vi "stop_device.vi"(8 "错误输入（无错误）":errorcluster) -> (0 "错误输出":errorcluster)   [LabVIEW 2013]
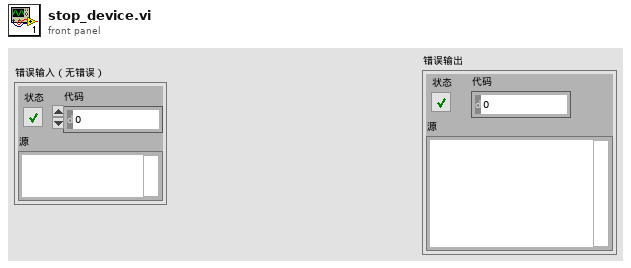
[diagram p1: front panel]
types:
  T1 = cluster{"cmd":string, "channel":i32, "value":dbl, "on/off":bool, "return value":refnum<vi>}
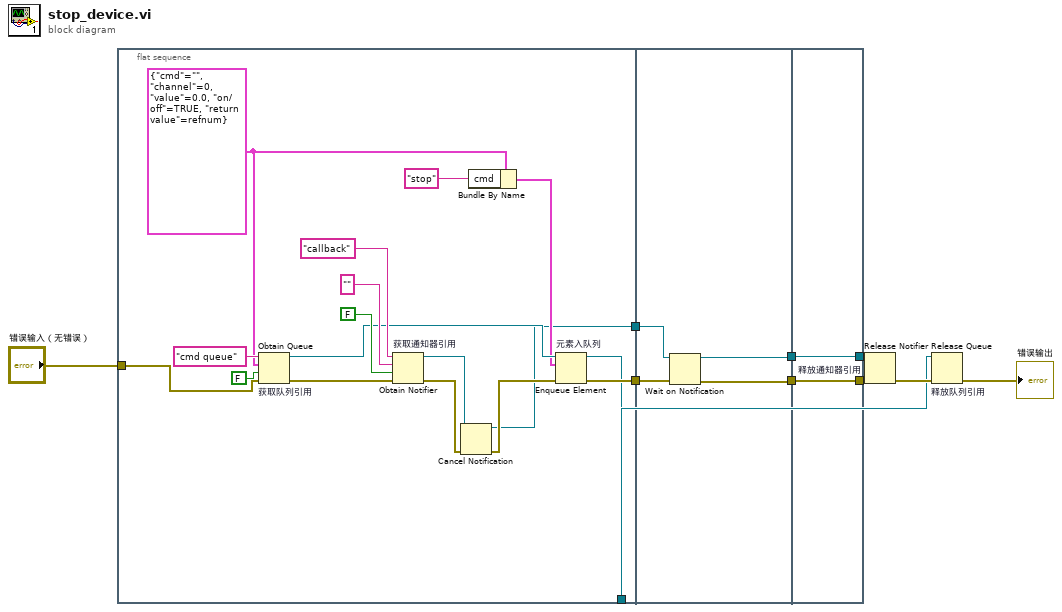
[diagram p0: block diagram]
diagram:
  n1 = flat-sequence {
    tunnel: [w11] -> w10
    tunnel: [w17] -> w5
    tunnel: [w16] -> w2
    tunnel: "错误输入（无错误）" -> [w15]
    tunnel: w10 -> [w31]
    tunnel: [w28] -> w9
    tunnel: [w29] -> w7
    tunnel: w5 -> [w30]
    tunnel: w9 -> [w33]
    tunnel: [w33] -> w8
    tunnel: w7 -> [w32]
    tunnel: [w32] -> w6
    frame #0 {
      w18 = T1 {"cmd"="", "channel"=0, "value"=0.0, "on/off"=TRUE, "return value"=refnum}
      n2 = Obtain Queue "获取队列引用"(name (unnamed)="cmd queue" ("名称（未命名）"), element data type=w18, create if not found? (T)=FALSE ("如未找到是否创建？(T)"), error in (no error)=w15) -> (queue out=w20:refnum<queue>, error out=w21:errorcluster)  [unwired: 1 in, 1 out]
      n3 = Obtain Notifier "获取通知器引用"(name (unnamed)="callback" ("名称（未命名）"), notification data type="", create if not found? (T)=FALSE ("如未找到是否创建？(T)"), error in (no error)=w21) -> (notifier out=w12:refnum<notifier>, error out=w14:errorcluster)  [unwired: 1 out]
      n4 = Cancel Notification(0:w12, 3:w14) -> (8:w11:refnum<notifier>, 11:w13:errorcluster)  [unwired: 1 out]
      n5 = Bundle By Name(cluster=w18, "cmd"="stop") -> (w19:T1)
      n6 = Enqueue Element "元素入队列"(queue=w20, element=w19, error in (no error)=w13) -> (queue out=w16:refnum<queue>, error out=w17:errorcluster)  [unwired: 1 in, 1 out]
    }
    frame #1 {
      n7 = Wait on Notification(notifier=w31, error in (no error)=w30) -> (notifier out=w28:refnum<notifier>, error out=w29:errorcluster)  [unwired: 2 in, 2 out]
    }
    frame #2 {
    }
  }
  n8 = Release Notifier "释放通知器引用"(notifier=w8, error in (no error)=w6) -> (error out=w4:errorcluster)  [unwired: 1 in, 2 out]
  n9 = Release Queue "释放队列引用"(queue=w2, error in (no error)=w4) -> (error out=→"错误输出":errorcluster)  [unwired: 1 in, 2 out]
